vi "Test AO.vi"() -> ()   [LabVIEW 2015]
uses:
  <vilib>/Platform/TimedLoop/XDataNode/timing_clust.ctl
  <vilib>/Platform/TimedLoop/XDataNode/nitl_modes.ctl
  <vilib>/Platform/TimedLoop/XDataNode/wakeup.ctl
  <vilib>/FPGAPlugInAG/cRIO-9081/niLvFpga_Open_cRIO-9081.vi
  <vilib>/Utility/error.llb/Error Cluster From Error Code.vi
  <vilib>/RVI Host/nirviSupport.llb/nirviErrorClusterFromErrorCode.vi
  <vilib>/rvi/errors/niLvFpgaAdjustHostInterfaceError.vi
  <vilib>/rvi/interface/common/niFpgaWaitOnOcc.vi
  <vilib>/FPGAPlugInAG/cRIO-9081/niLvFpga_Close_cRIO-9081.vi
  FPGA Ref.ctl
  <vilib>/rvi/interface/nirviOpenFPGA/nirviOpenFPGA.xnode
  FPGA Bitfiles/Nicholas.lvbitx
  <vilib>/rvi/interface/nirviMethod/nirviMethod.xnode
  <vilib>/Platform/TimedLoop/XDataNode/XDataNode.xnode
  <vilib>/rvi/interface/nirviReadWriteControl/nirviReadWriteControl.xnode
  <vilib>/rvi/interface/nirviCloseFPGA/nirviCloseFPGA.xnode
  <vilib>/Platform/TimedLoop/XDataNode/XDNodeRunTimeDep.lvlib
  NiFpgaLv.dll
  <vilib>/FPGAPlugInAG/cRIO-9081/niLvFpga_ConfigureFifo_cRIO-9081.vi
  <vilib>/rvi/errors/niLvFpgaMergeErrorWithErrorCode.vi
  <vilib>/FPGAPlugInAG/cRIO-9081/niLvFpga_StartFifo_cRIO-9081.vi
  <vilib>/rvi/interface/nirviMethod/StockFPGA_InlinedMethodWaitForSingleIRQ.vi
  <vilib>/FPGAPlugInAG/cRIO-9081/niLvFpga_WaitOnIrq_cRIO-9081.vi
  <vilib>/FPGAPlugInAG/cRIO-9081/niLvFpga_AcknowledgeIrq_cRIO-9081.vi
  <vilib>/FPGAPlugInAG/cRIO-9081/niLvFpga_WriteFifo_cRIO-9081.vi
  <vilib>/FPGAPlugInAG/cRIO-9081/niLvFpga_ReadFifo_cRIO-9081.vi
panel:
  out "sOffset":fxp<+/-,16,16>
  out "sRange":fxp<+,32,0>
  in  "Duty Cycle":fxp<+,32,0>
  out "Waveform Graph":i16[](graph)
  in  "Speaker":cluster{"Vscale":fxp<+,32,1>, "Offset":i16}
  out "error out":errorcluster
  in  "Spk?":bool
  in  "Mod":enum16{"Sine", "Square"}(ring)
  in  "Vrange":dbl=0.165 format="%#_13g"
  in  "offset":dbl=0.165 format="%#_13g"
  in  "Stop":bool
  in  "F":dbl
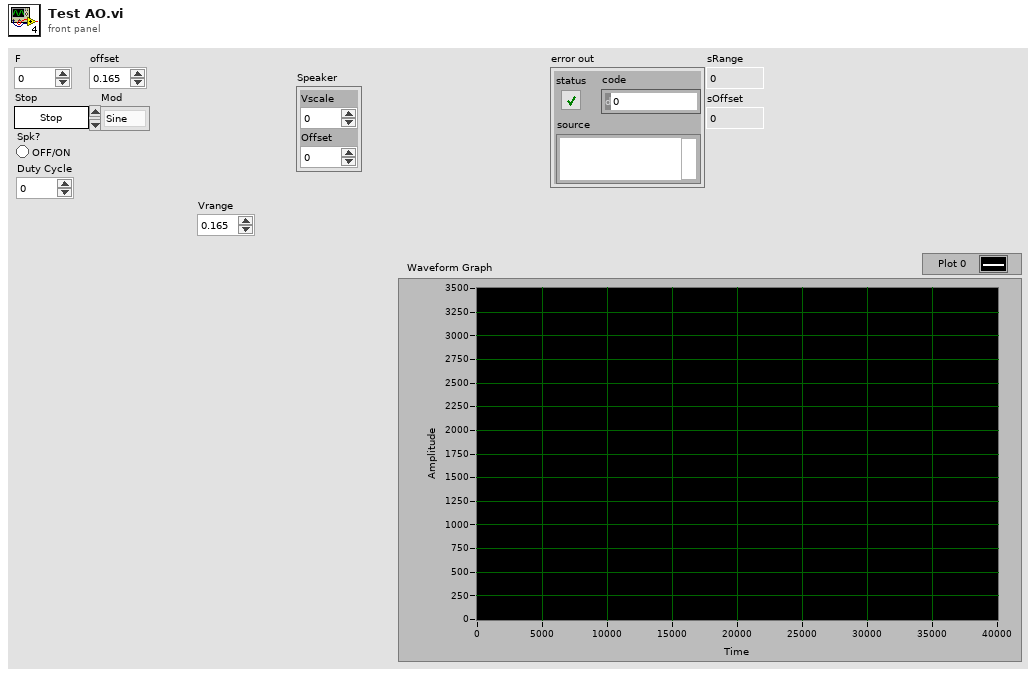
[diagram p1: front panel]
types:
  T1 = typedef "FPGA Ref.ctl" = refnum<k20>
  T2 = typedef "XDNodeRunTimeDep.lvlib/timing_clust.ctl" = cluster{"Expected End [f-1]":u64, "Actual End [f-1]":u64, "Finished Late? [f-1]":bool, "Expected End [i-1]":u64, "Actual End [i-1]":u64, "Finished Late? [i-1]":bool, "Expected Start [i]":u64, "Actual Start [i]":u64, "Expected Start [f]":u64, "Actual Start [f]":u64, "Source Name":string, "Structure Name":string, "Period":i64, "Deadline":i64, "Offset":i64, "Start":i64, "Priority":i32, "Timeout":i32, "Mode":T3, "Wakeup Reason":T4, "Error":errorcluster, "Source Type":string, "Secondary Source Type":string, "Global End Time":u64, "Global Start Time":u64, "Frame Duration":u64, "Iteration Duration":u64, "Assigned CPU":i32, "I/O Scan Engine Mode":u32}
  T3 = typedef "XDNodeRunTimeDep.lvlib/nitl_modes.ctl" = enum32{"No Change", "Process missed periods, maintain original phase", "Discard missed periods, maintain original phase", "Process missed periods, ignore original phase", "Discard missed periods, ignore original phase"}
  T4 = typedef "XDNodeRunTimeDep.lvlib/wakeup.ctl" = enum32{"Normal", "Aborted", "Asynchronous wakeup", "Timing source error", "Timed loop error", "Timeout"}
  T5 = cluster{"f0":fxp<+,32,0>, "Mod":enum16{"Sine", "Square"}, "Vscale":fxp<+,32,0>, "Offset":i16}
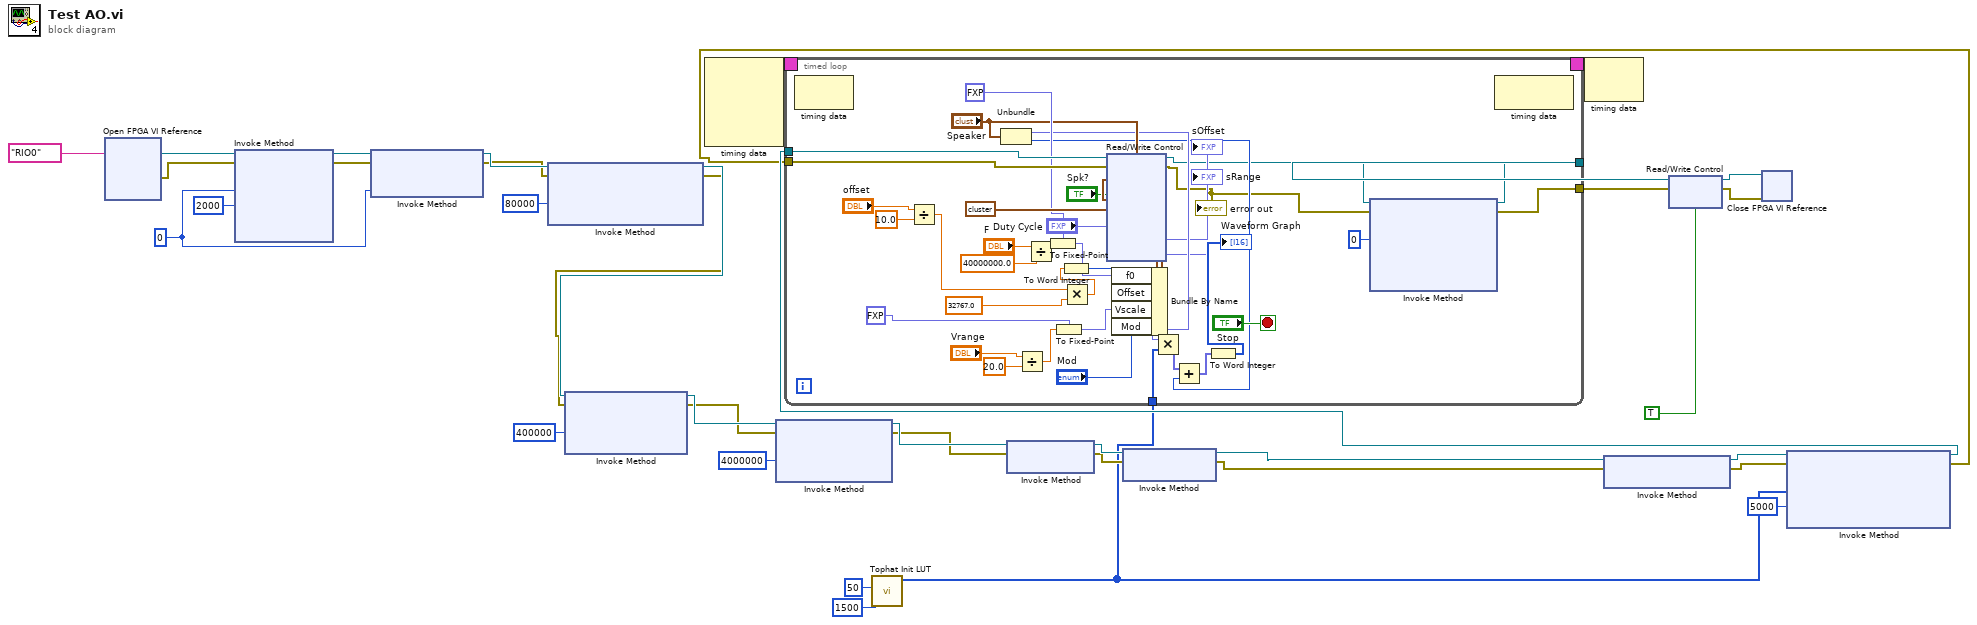
[diagram p0: block diagram]
diagram:
  w33 = 0 ("IRQ Number(s)")
  n1 = xnode "Open FPGA VI Reference"("resource name"=tag "RIO0") -> ("FPGA VI Reference Out"=w32:T1, "error out"=w31:errorcluster)  [unwired: 1 in]
  n2 = xnode "Invoke Method"("FPGA VI Reference In"=w32, "error in"=w31, "IRQ Number(s)"=w33, "Timeout (ms)"=2000) -> ("FPGA VI Reference Out"=w35:T1, "error out"=w34:errorcluster)  [unwired: 2 out]
  n3 = xnode "Invoke Method"("FPGA VI Reference In"=w35, "error in"=w34, "IRQ Number(s)"=w33) -> ("FPGA VI Reference Out"=w23:T1, "error out"=w19:errorcluster)
  n4 = xnode "Invoke Method"("FPGA VI Reference In"=w23, "error in"=w19, "Requested Depth"=u32 80000) -> ("FPGA VI Reference Out"=w20:T1, "error out"=w18:errorcluster)  [unwired: 1 out]
  n5 = xnode "Invoke Method"("FPGA VI Reference In"=w20, "error in"=w18, "Requested Depth"=u32 400000) -> ("FPGA VI Reference Out"=w17:T1, "error out"=w16:errorcluster)  [unwired: 1 out]
  n6 = node-c288() -> (w30:T2)  [unwired: 4 in]
  n7 = xnode "Invoke Method"("FPGA VI Reference In"=w17, "error in"=w16, "Requested Depth"=u32 4000000) -> ("FPGA VI Reference Out"=w14:T1, "error out"=w13:errorcluster)  [unwired: 1 out]
  n8 = call "Tophat Init LUT.vi"("Df"=i16 50, "f0"=i16 1500) -> ("Init Data Out"=w1:i16[])  [unwired: 7 in]
  n9 = xnode "Invoke Method"("FPGA VI Reference In"=w14, "error in"=w13) -> ("FPGA VI Reference Out"=w12:T1, "error out"=w11:errorcluster)
  n10 = xnode "Invoke Method"("FPGA VI Reference In"=w12, "error in"=w11) -> ("FPGA VI Reference Out"=w10:T1, "error out"=w9:errorcluster)
  n11 = xnode "Invoke Method"("FPGA VI Reference In"=w10, "error in"=w9) -> ("FPGA VI Reference Out"=w8:T1, "error out"=w7:errorcluster)
  n12 = xnode "Invoke Method"("FPGA VI Reference In"=w8, "error in"=w7, "Data"=w1, "Timeout (ms)"=5000) -> ("FPGA VI Reference Out"=w5:T1, "error out"=w4:errorcluster)  [unwired: 1 out]
  n13 = timed-loop {
    tunnel: w5 -> [w75]
    tunnel: w4 -> [w74]
    timing: w30 -> [_]
    timing-out: [_] -> w29
    tunnel: [w39] -> w27
    tunnel: [w38] -> w26
    tunnel: w1 -> [w51]
    stop <- "Stop" stop-if-true
    n14 = node-c288() -> ()  [unwired: 1 in, 1 out]
    n15 = Divide(x="offset", y=10.0) -> (x/y=w65:dbl)
    n16 = Unbundle("Speaker") -> ("Vscale"=w49:fxp<+,32,1>, "Offset"=w47:i16)
    n17 = Divide(x="Vrange", y=20.0) -> (x/y=w54:dbl)
    n18 = Divide(x="F", y=40000000.0) -> (x/y=w60:dbl)
    n19 = To Fixed-Point(fixed-point type=fxp<+,32,0> 0.0 ("f0"), number=w60) -> (fixed-point=w59:fxp<+,32,0>)
    n20 = To Fixed-Point(fixed-point type=fxp<+,32,0> 0.0 ("Vscale"), number=w54) -> (fixed-point=w53:fxp<+,32,0>)
    n21 = Multiply(x=w65, y=32767.0 ("Offset")) -> (x*y=w56:dbl)
    n22 = To Word Integer(number=w56) -> (16bit integer=w57:i16)
    n23 = Bundle By Name(cluster=T5 {"f0"=0.0, "Mod"=enum."Sine", "Vscale"=0.1650000000372529, "Offset"=0} ("Wave"), "f0"=w59, "Offset"=w57, "Vscale"=w53, "Mod"="Mod") -> (w70:T5)
    n24 = xnode "Read/Write Control"("FPGA VI Reference In"=w75, "error in"=w74, "Wave"=w70, "Spk?"="Spk?", "Speaker"="Speaker", "pDC"="Duty Cycle") -> ("FPGA VI Reference Out"=w42:T1, "error out"=w41:errorcluster, "sRange"=→"sRange":fxp<+,32,0>, "sOffset"=→"sOffset":fxp<+/-,16,16>)
    "error out" <- w41
    n25 = Multiply(x=w49, y=w51) -> (x*y=w48:fxp<+/-,48,17>[])
    n26 = Add(x=w48, y=w47) -> (x+y=w46:fxp<+/-,49,18>[])
    n27 = To Word Integer(number=w46) -> (16bit integer=→"Waveform Graph":i16[])
    n28 = xnode "Invoke Method"("FPGA VI Reference In"=w42, "error in"=w41, "Number of Elements"=u32 0) -> ("FPGA VI Reference Out"=w39:T1, "error out"=w38:errorcluster)  [unwired: 1 in, 2 out]
    n29 = node-c288() -> ()  [unwired: 1 in, 1 out]
  }
  n30 = node-c288(w29) -> ()  [unwired: 1 out]
  n31 = xnode "Read/Write Control"("FPGA VI Reference In"=w27, "error in"=w26, "Stop"=TRUE) -> ("FPGA VI Reference Out"=w25:T1, "error out"=w24:errorcluster)
  n32 = xnode "Close FPGA VI Reference"("FPGA VI Reference In"=w25, "error in"=w24) -> ()  [unwired: 1 out]
